vi "OutputPicture.vi"(6 "像素大小":cluster{"x":i32, "y":i32}, 7 "显示起点":cluster{dbl, dbl}, 8 "backcolor":u32(colorbox)=16777215, 9 "color":u32(colorbox), 11 "二维码":bool[][](array[boolean])) -> (3 "new picture":picture caption="新图片")   [LabVIEW 2016, in "opSignIn.lvlib"]
uses:
  opSignIn.lvlib
panel:
  out "empty picture":picture caption="空图片"
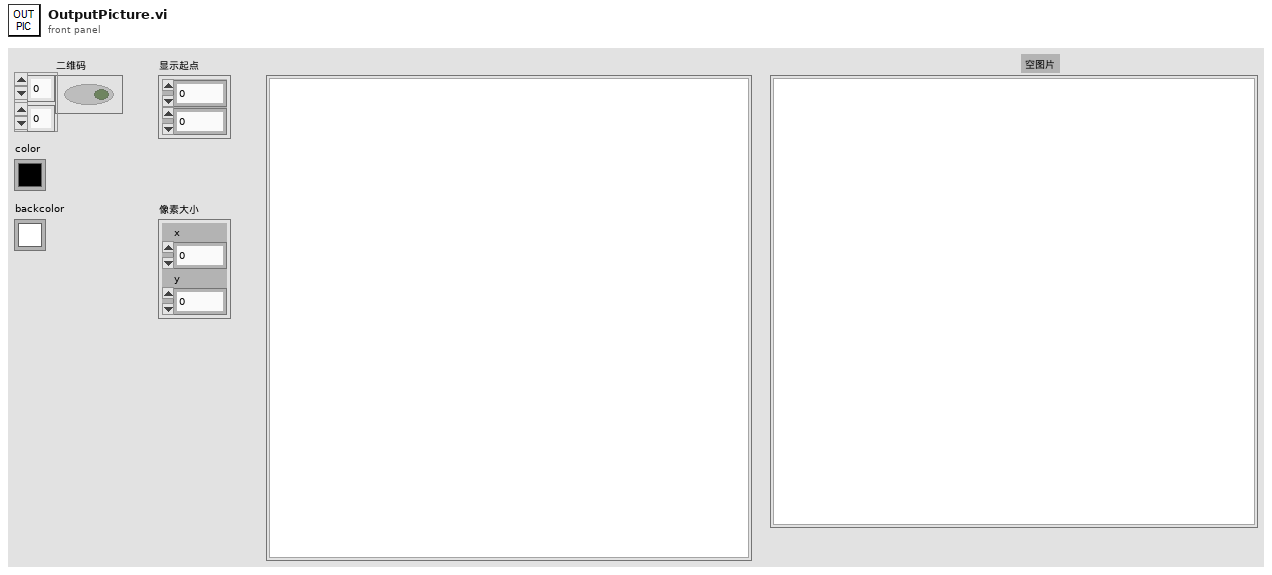
[diagram p1: front panel]
types:
  T1 = cluster{"Width":i16, "Style":enum32{"Solid", "Dash", "Dot", "DashDot", "DashDotDot"}}
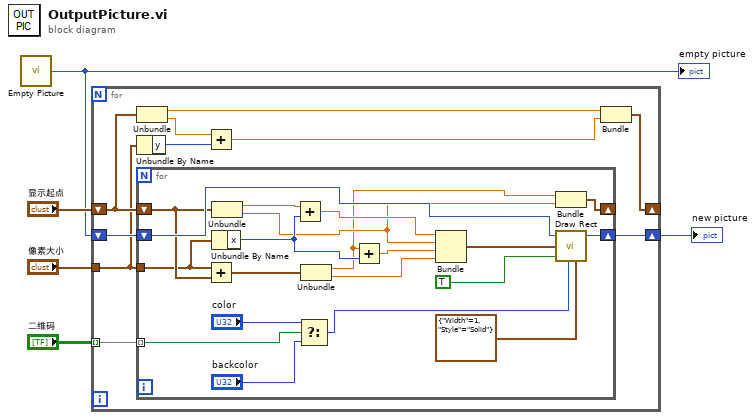
[diagram p0: block diagram]
diagram:
  n1 = call "Empty Picture"() -> ("empty picture"=w2:picture)
  "empty picture" <- w2
  n2 = for {
    shift-right: [w14] -> _
    shift-left: "显示起点" -> [w13]
    shift-right: [w11] -> w3
    shift-left: w2 -> [w12]
    tunnel: "像素大小" -> [w10]
    tunnel: "二维码" -> [w6] mode=indexing
    n3 = Unbundle(w13) -> (w15:dbl, w7:dbl)
    n4 = Unbundle By Name(w10) -> ("y"=w9:i32)
    n5 = for {
      shift-right: [w23] -> _
      shift-left: w13 -> [w21]
      shift-right: [w22] -> w11
      shift-left: w12 -> [w33]
      tunnel: w10 -> [w19]
      tunnel: w6 -> [w16] mode=indexing
      n6 = Add(x=w19, y=w21) -> (x+y=w20:cluster{dbl, dbl})
      n7 = Unbundle(w21) -> (w32:dbl, w18:dbl)
      n8 = Unbundle By Name(w19) -> ("x"=w30:i32)
      n9 = Add(x=w32, y=w30) -> (x+y=w31:dbl)
      n10 = Select(t="color", s=w16, f="backcolor") -> (s? t:f=w26:u32)
      n11 = Unbundle(w20) -> (w17:dbl, w24:dbl)
      n12 = Add(x=w17, y=w30) -> (x+y=w25:dbl)
      n13 = Bundle(w31, w18, w25, w24) -> (w29:cluster{dbl, dbl, dbl, dbl})  [unwired: 1 in]
      n14 = Bundle(w17, w18) -> (w23:cluster{dbl, dbl})  [unwired: 1 in]
      n15 = call <vilib>:"Draw Rect.vi"("picture"=w33, "rect"=w29, "fill?(F)"=TRUE, "color(black)"=w26, "pen"=T1 {"Width"=1, "Style"=enum."Solid"}) -> ("new picture"=w22:picture)  [unwired: 4 in]
    }
    n16 = Add(x=w7, y=w9) -> (x+y=w8:dbl)
    n17 = Bundle(w15, w8) -> (w14:cluster{dbl, dbl})  [unwired: 1 in]
  }
  "new picture" <- w3
